vi "Image Collector.vi"(8 "error in (no error)":errorcluster) -> (0 "error out":errorcluster)   [LabVIEW 2014]
uses:
  <vilib>/vision/driver/IMAQdx.llb/IMAQdx Buffer Number Mode.ctl
  ImageCluster.ctl
  <vilib>/vision/Image Controls.llb/IMAQ Image.ctl
  Globals.vi
  <vilib>/vision/driver/NI_Vision_Acquisition_Software.lvlib
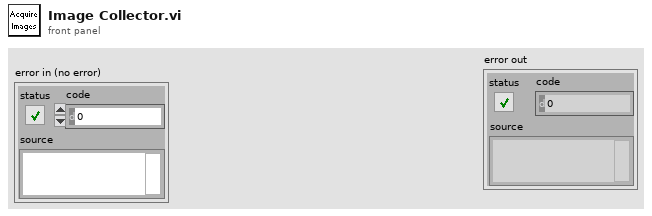
[diagram p1: front panel]
types:
  T1 = typedef "ImageCluster.ctl" = cluster{"Screenshot":T2, "Time (s)":dbl}
  T2 = typedef "IMAQ Image.ctl" = refnum<image>
  T3 = typedef "NI_Vision_Acquisition_Software.lvlib/IMAQdx Buffer Number Mode.ctl" = enum32{"Next", "Last", "Buffer Number"}
  T4 = typedef "Image Type" = u32
  T5 = typedef "IMAQdx.ctl" = refnum<k21>
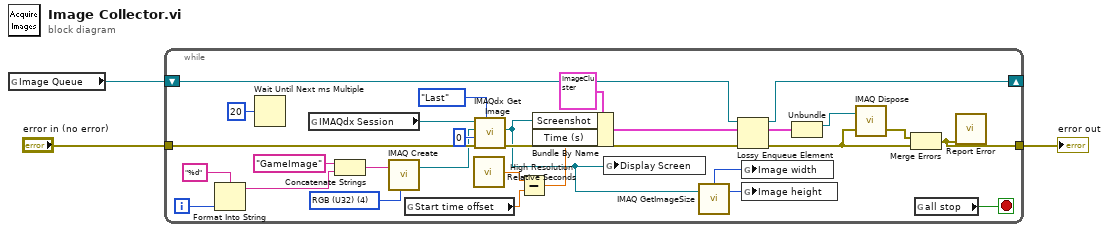
[diagram p0: block diagram]
diagram:
  n1 = global read "Globals.vi" "Image Queue"() -> (w3:refnum<queue>)
  n2 = while {
    shift-right: [w23] -> _
    shift-left: w3 -> [w24]
    tunnel: "error in (no error)" -> [w32]
    tunnel: [w5] -> w1
    i -> [w13]
    stop <- w9 stop-if-true
    w17 = T4 4 items=["Grayscale (U8)", "Grayscale (I16)", "Grayscale (SGL)", "Complex (CSG)", "RGB (U32)", "HSL (U32)", "RGB (U64)", "Grayscale (U16)"] ("Image Type")
    n3 = Format Into String(format string="%d", w13) -> (resulting string=w14:string)  [unwired: 2 in, 1 out]
    n4 = Wait Until Next ms Multiple(millisecond multiple=u32 20) -> ()  [unwired: 1 out]
    n5 = global read "Globals.vi" "IMAQdx Session"() -> (w22:T5)
    n6 = Concatenate Strings("GameImage" ("string"), w14) -> (w16:string)
    n7 = call "IMAQ Create"("Image Name"=w16, "Image Type"=w17) -> ("New Image"=w18:T2)  [unwired: 3 in, 1 out]
    n8 = global read "Globals.vi" "Start time offset"() -> (w8:dbl)
    n9 = call <vilib>:"High Resolution Relative Seconds.vi"() -> ("relative seconds"=w26:dbl)
    n10 = call <vilib>:"IMAQdx Get Image.vi"("Buffer Number Mode (Next)"=IMAQdx_Buffer_Number_Mode."Last", "error in"=w32, "Buffer Number In"=u32 0, "Image In"=w18, "Session In"=w22) -> ("error out"=w27:errorcluster, "Image Out"=w19:T2)  [unwired: 3 in, 2 out]
    n11 = Subtract(x=w26, y=w8) -> (x-y=w25:dbl)
    n12 = Bundle By Name(cluster=T1 {"Screenshot"=refnum, "Time (s)"=0.0}, "Screenshot"=w19, "Time (s)"=w25) -> (w28:T1)
    n13 = global write "Globals.vi" "Display Screen"(w19) -> ()
    n14 = call "IMAQ GetImageSize"("Image"=w19) -> ("Y Resolution"=w20:i32, "X Resolution"=w21:i32)  [unwired: 3 in, 1 out]
    n15 = Lossy Enqueue Element(queue=w24, element=w28, error in (no error)=w27) -> (queue out=w23:refnum<queue>, overflow element=w11:T1, error out=w6:errorcluster)  [unwired: 1 out]
    n16 = global write "Globals.vi" "Image width"(w21) -> ()
    n17 = global write "Globals.vi" "Image height"(w20) -> ()
    n18 = Unbundle(w11) -> ("Screenshot"=w10:T2)  [unwired: 1 out]
    n19 = call "IMAQ Dispose"("Image"=w10, "error in (no error)"=w6) -> ("error out"=w7:errorcluster)  [unwired: 4 in]
    n20 = Merge Errors(w7, w6) -> (w5:errorcluster)
    n21 = global read "Globals.vi" "all stop"() -> (w9:bool)
    n22 = call "Report Error.vi"("error in (no error)"=w5) -> ()  [unwired: 11 in]
  }
  "error out" <- w1
